vi "write_acq_time.vi"(8 "error in (no error)":errorcluster, 10 "acq_time":i32, 11 "hydraharp in":refnum<class "hydraharp.lvclass">) -> (0 "error out":errorcluster, 3 "hydraharp out":refnum<class "hydraharp.lvclass">)   [LabVIEW 2015, in "hydraharp.lvclass"]
uses:
  hydraharp.lvclass
  hydraharp.lvclass/hydraharp.ctl
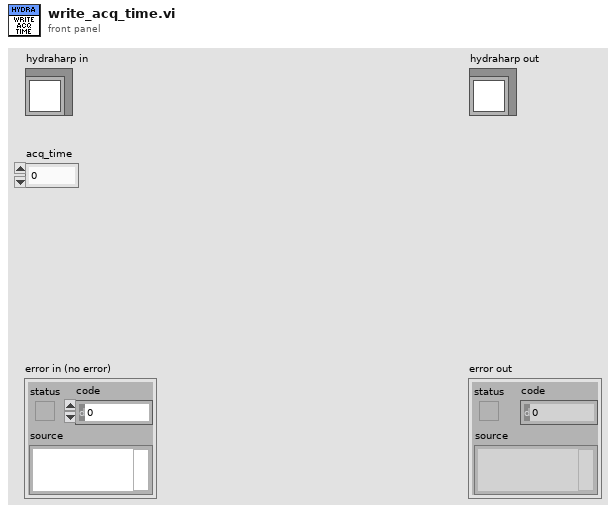
[diagram p1: front panel]
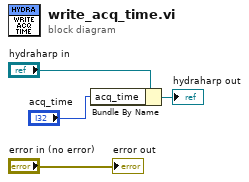
[diagram p0: block diagram]
diagram:
  n1 = Bundle By Name(cluster="hydraharp in", "acq_time"="acq_time") -> (→"hydraharp out":refnum<class "hydraharp.lvclass">)
  "error out" <- "error in (no error)"
